vi "niRFSTS DCPower Measure.vi"(8 "Published Data Id":string="Total DC Current (A)", 9 "Aperture Time":dbl=0.001 format="%#_6p", 10 "Pins":string[](array[string]), 11 "Semiconductor Module Context":T1) -> (0 "error out":errorcluster)   [LabVIEW 2014]
uses:
  <vilib>/NI_TestStand_SemiconductorModule/NI_TestStand_Semiconductor_Module.lvlibp/PinMap/General/SemiconductorModuleContext.ctl
  <instrlib>/niDCPower/nidcpower.llb/niDCPower Measurement Type.ctl
  <vilib>/NI_TestStand_SemiconductorModule/NI_TestStand_Semiconductor_Module.lvlibp/PinMap/DC Power/PinsToNIDCPowerSessions.vi
  <vilib>/NI_TestStand_SemiconductorModule/NI_TestStand_Semiconductor_Module.lvlibp/PinMap/General/Publish/PublishDataDoubleFunctionalTest.vi
  <vilib>/NI_TestStand_SemiconductorModule/NI_TestStand_Semiconductor_Module.lvlibp
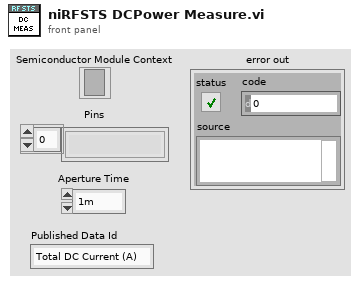
[diagram p1: front panel]
types:
  T1 = typedef "NI_TestStand_Semiconductor_Module.lvlibp/SemiconductorModuleContext.ctl" = refnum<k7>
  T2 = typedef "niDCPower Measurement Type.ctl" = i32
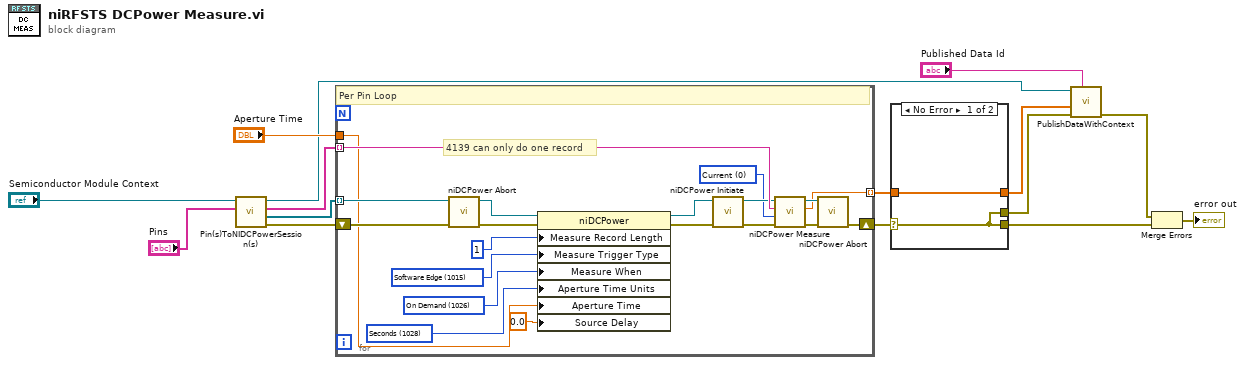
[diagram p0: block diagram]
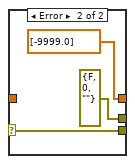
[diagram p2: hidden frame]
diagram:
  n1 = call-poly <vilib>:"Pin(s)ToNIDCPowerSession(s).vi"("Pins"="Pins", "Semiconductor Module Context"="Semiconductor Module Context") -> ("error out"=w9:errorcluster, "Instrument Sessions"=w13:refnum<k15>[], "Channel Lists"=w12:string[], "Semiconductor Module Context Out"=w8:T1)  [unwired: 5 in, 1 out]
  n2 = for {
    tunnel: w13 -> [w32] mode=indexing
    tunnel: w12 -> [w31] mode=indexing
    tunnel: "Aperture Time" -> [w30]
    tunnel: [w17] -> w5 mode=indexing
    shift-right: [w20] -> w7
    shift-left: w9 -> [w33]
    w16 = T2 0 items=["Current", "Voltage"] ("measurement type")
    w26 = 1026 items=["Automatically after Source Complete"=1025, "On Demand"=1026, "On Measure Trigger"=1027] ("Measure When")
    w27 = 1028 items=["Seconds"=1028, "Power Line Cycles"=1029] ("Measurement:Aperture Time Units")
    w28 = 1015 items=["Digital Edge"=1014, "Software Edge"=1015, "None"=1012] ("Triggers:Measure Trigger:Trigger Type")
    # "4139 can only do one record"
    # "Per Pin Loop"
    n3 = call <instrlib>:"niDCPower Abort.vi"("error in (no error)"=w33, "instrument handle"=w32) -> ("error out"=w34:errorcluster, "instrument handle out"=w35:refnum<k15>)  [unwired: 8 in]
    n4 = property class="niDCPower"(reference=w35, error in=w34, "Measure Record Length"=1 ("Measurement:Measure Record Length"), "Measure Trigger Type"=w28, "Measure When"=w26, "Aperture Time Units"=w27, "Aperture Time"=w30, "Source Delay"=0.0 ("Source:Advanced:Source Delay")) -> (reference out=w24:refnum<k15>, error out=w25:errorcluster)
    n5 = call <instrlib>:"niDCPower Initiate.vi"("error in (no error)"=w25, "instrument handle"=w24) -> ("error out"=w18:errorcluster, "instrument handle out"=w19:refnum<k15>)  [unwired: 8 in]
    n6 = call <instrlib>:"niDCPower Measure.vi"("error in (no error)"=w18, "measurement type"=w16, "channel name"=w31, "instrument handle"=w19) -> ("error out"=w21:errorcluster, "measurement"=w17:dbl, "instrument handle out"=w22:refnum<k15>)  [unwired: 5 in]
    n7 = call <instrlib>:"niDCPower Abort.vi"("error in (no error)"=w21, "instrument handle"=w22) -> ("error out"=w20:errorcluster)  [unwired: 8 in, 1 out]
  }
  n8 = case shown="No Error" w7 {
    selector: w7 -> [w37 w39]
    tunnel: w5 -> [w36 _]
    tunnel: [w36 dbl[] [-9999.0]] -> w4
    tunnel: [w37 errorcluster {"status"=FALSE, "code"=0, "source"=""} ("error IO")] -> w6
    tunnel: [w37 w39] -> w2
    frame No Error {
    }
    frame Error {
    }
  }
  n9 = call-poly <vilib>:"PublishDataWithContext.vi"("Published Data Id"="Published Data Id", "error in (no error)"=w6, "Data In"=w4, "Semiconductor Module Context"=w8) -> ("error out"=w3:errorcluster)  [unwired: 6 in, 1 out]
  n10 = Merge Errors(w3, w2) -> (→"error out":errorcluster)
